vi "Write Hardware.lvlib_CCD.lvlib_CCD.lvclass.vi"(8 "error in (no error)":errorcluster, 10 "Hardware.lvlib:CCD.lvlib:CCD.lvclass":refnum<class "CCD.lvclass">, 11 "CCD Configuration in":refnum<class "CCD Configuration.lvclass">) -> (0 "error out":errorcluster, 3 "CCD Configuration out":refnum<class "CCD Configuration.lvclass">)   [LabVIEW 2016, in "CCD.lvlib" / "CCD Configuration.lvclass"]
uses:
  <userlib>/Common Components/Hardware/CCD/CCD Configuration.lvclass
  <userlib>/Common Components/Hardware/CCD/CCD/CCD.lvclass
  <userlib>/Common Components/Hardware/CCD/CCD Configuration.lvclass/CCD Configuration.ctl
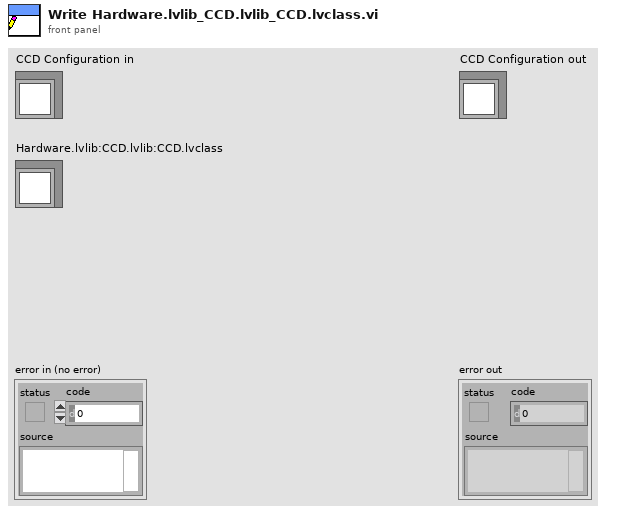
[diagram p1: front panel]
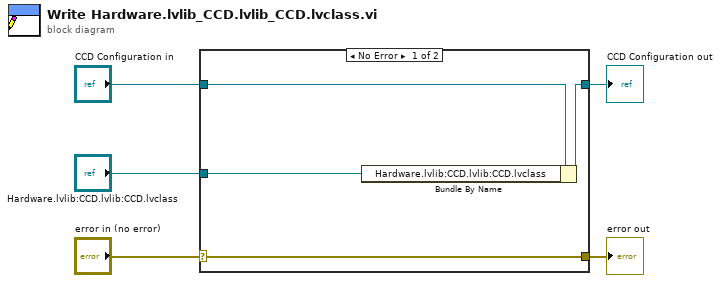
[diagram p0: block diagram]
diagram:
  n1 = case shown="No Error" "error in (no error)" {
    selector: "error in (no error)" -> [w9 w10]
    tunnel: [w9 w10] -> w4
    tunnel: [w7 w11] -> w2
    tunnel: "CCD Configuration in" -> [w8 w11]
    tunnel: "Hardware.lvlib:CCD.lvlib:CCD.lvclass" -> [w6 _]
    frame No Error {
      n2 = Bundle By Name(cluster=w8, "Hardware.lvlib:CCD.lvlib:CCD.lvclass"=w6) -> (w7:refnum<class "CCD Configuration.lvclass">)
    }
    frame Error {
    }
  }
  "error out" <- w4
  "CCD Configuration out" <- w2
